vi "Vision Research Phantom Series PhFile PhMeasureCineWB.vi"(0 "hC in":u32=1, 1 "pP":T3, 2 "SquareSide":i32, 3 "pRng":T1, 5 "Error In (no error)":errorcluster) -> (14 "hC out":u32=1, 16 "pWB":T2, 17 "pSatCnt":u32, 19 "Error Out":errorcluster)   [LabVIEW 2013, in "VRI.lvlib"]
doc: "PhFile.dll\n\nPhMeasureCineWB\nHRESULT PhMeasureCineWB(CINEHANDLE hC, PPOINT pP, int SquareSide, PIMRANGE pRng,\nPWBGAIN pWB, PUINT pSatCnt)\n\nParameters Description\nhC (in) Handle of the cine.\npP (in) Point, center of the square where to do the average.\nSquareSide (in) SquareSide where to average the pixels.\npRng (in) Range of images from the cine to average.\npWB (out) Result: WBGAIN, the compensating gains on red and blue.\npSatCnt (out) Result: saturated pixels count; an indication about how correct\n the measurement is. To obtain best results, avoid having saturated \n pixels in the square used for this measurement. It can be NULL if\n not needed.\nReturn HRESULT (0 = Ok)\nComments Finds the pixel component averages around a point in a given cine file.\n Use an internal call to PhComputeWB to prepare the WBGAIN\n compensation factors and count of the saturated pixels in the\n specified area. s"
uses:
  VRI.lvlib
  _Type Defs/Point.ctl
  _Type Defs/PhInt WBGAIN.ctl
  _Type Defs/PHCon IMRANGE.ctl
  Phantom DLLs/PhFile.Dll
panel:
  # "For instructions on the use of this VI, press Ctrl+H to display the help window and move the mouse over the icon, controls, and indicators"
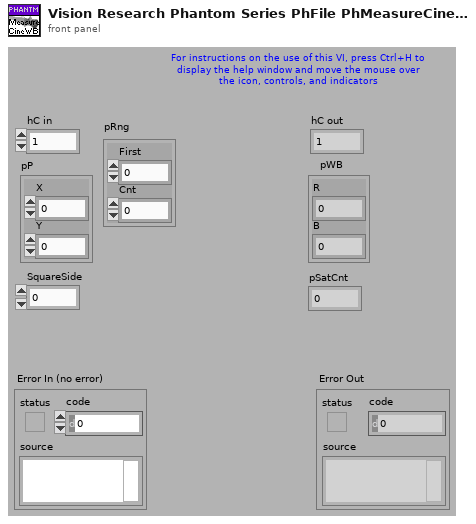
[diagram p1: front panel]
types:
  T1 = typedef "VRI.lvlib/PHCon IMRANGE.ctl" = cluster{"First":i32, "Cnt":u32}
  T2 = typedef "VRI.lvlib/PhInt WBGAIN.ctl" = cluster{"R":sgl, "B":sgl}
  T3 = typedef "VRI.lvlib/Point.ctl" = cluster{"X":i32, "Y":i32}
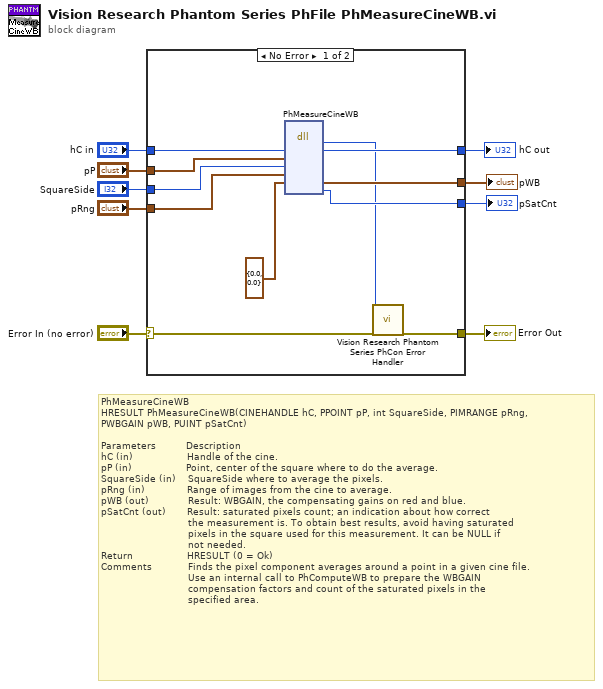
[diagram p0: block diagram]
diagram:
  # "PhMeasureCineWB\nHRESULT PhMeasureCineWB(CINEHANDLE hC, PPOINT pP, int SquareSide, PIMRANGE pRng,\nPWBGAIN pWB, PUINT pSatCnt)\n\nParameters          Description\nhC (in)                  Handle of the cine.\npP (in)                  Point, center of the square where to do the average.\nSquareSide (in)    SquareSide where to average the pixels.\npRng (in)              Range of images from the cine to average.\npWB (out)             Result: WBGAIN, the compensating gains on red and blue.\npSatCnt (out)       Result: saturated pixels count; an indication about how correct\n                             the measurement is. To obtain best results, avoid having saturated \n                             pixels in the square used for this measurement. It can be NULL if\n                             not needed.\nReturn                  HRESULT (0 = Ok)\nComments            Finds the pixel component averages around a point in a given cine file.\n                             Use an internal call to PhComputeWB to prepare the WBGAIN\n                             compensation factors and count of the saturated pixels in the\n                             specified area."
  n1 = case shown="No Error" "Error In (no error)" {
    selector: "Error In (no error)" -> [w20 w22]
    tunnel: [w19 w22] -> w8
    tunnel: "hC in" -> [w18 w21]
    tunnel: [w17 w21] -> w6
    tunnel: "pP" -> [w16 _]
    tunnel: "SquareSide" -> [w15 _]
    tunnel: [w14 _] -> w3
    tunnel: [w13 _] -> w2
    tunnel: "pRng" -> [w12 _]
    frame No Error {
      n2 = dll-call lib="C:/Projects/SDK/64-bit/Vision Research Phantom Series Labview Driver/Phantom DLLs/PhFile.dll" fn="PhMeasureCineWB"("hC"=w18, "pP"=w16, "SquareSide"=w15, "pRng"=w12, "pWB"=T2 {"R"=0.0, "B"=0.0} ("pWB 2")) -> ("HRESULT"=w11:i32, "hC"=w17:u32, "pWB"=w14:T2, "pSatCnt"=w13:u32)  [unwired: 6 in, 3 out]
      n3 = call "Vision Research Phantom Series PhCon Error Handler.vi"("ErrNo"=w11, "Error In (no error)"=w20) -> ("Error Out"=w19:errorcluster)  [unwired: 17 out]
    }
    frame Error {
    }
  }
  "Error Out" <- w8
  "hC out" <- w6
  "pSatCnt" <- w2
  "pWB" <- w3
